vi "Library Time.vi"() -> (0 "time":dbl format="%<%H:%M:%S\n%Y/%m/%d>T")   [LabVIEW 2012]
doc: "This VI can be replaced with a customized time source. By using it consistently throughout an application, you will need to modify only this one VI to switch time sources. Its default implementation simply returns the system time using the LabVIEW get date/time in seconds function. An alternate implementation should stick to the same epoch (1-Jan-1904, 12:00AM) and scaling (seconds)."
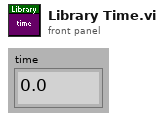
[diagram p1: front panel]
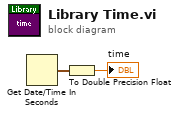
[diagram p0: block diagram]
diagram:
  n1 = Get Date/Time In Seconds() -> (seconds since 1Jan1904=w1:timestamp)
  n2 = To Double Precision Float(number=w1) -> (double precision float=→"time":dbl)
